vi "Process Flushed Data.vi"(8 "error in":errorcluster, 10 "Flushed elements":T1[](array[typedef]), 11 "Report Generator in":refnum<class "Report Generator.lvclass">) -> (0 "error out":errorcluster, 3 "Report Generator out":refnum<class "Report Generator.lvclass">)   [LabVIEW 2019, in "Report Generator.lvlib" / "Report Generator.lvclass"]
uses:
  Library/Report Generator.lvclass
  C:/Users/Public/Documents/Development/builds/Engine/Engine.lvlibp/Project/Engine.lvclass
  builds/Tools/QDMH.lvlibp/Custom Controls/QDMH Message.ctl
  Library/Report Generator.lvclass/Report Generator.ctl
  builds/Tools/Report.lvlibp/Custom Controls/Report Action.ctl
  builds/Tools/Report.lvlibp/Report.lvclass
  builds/Engine/Engine.lvlibp/Accessors/Read Directory.vi
  builds/Tools/Report.lvlibp/Accessors/Read Open.vi
  builds/Engine/Engine.lvlibp/Accessors/Write Directory.vi
  builds/Tools/QDMH.lvlibp/QDMH.lvclass
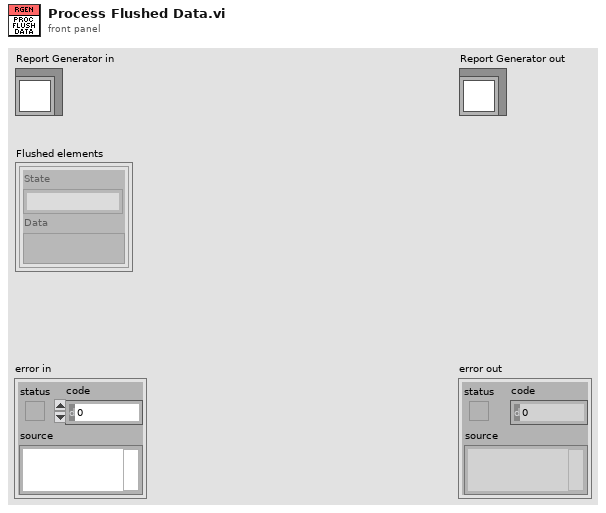
[diagram p1: front panel]
types:
  T1 = typedef "QDMH.lvlibp/QDMH.lvclass/QDMH Message.ctl" = cluster{"State":string, "Data":variant}
  T2 = typedef "Report.lvlibp/Report.lvclass/Report Action.ctl" = enum16{"Create", "Append", "Destroy"}
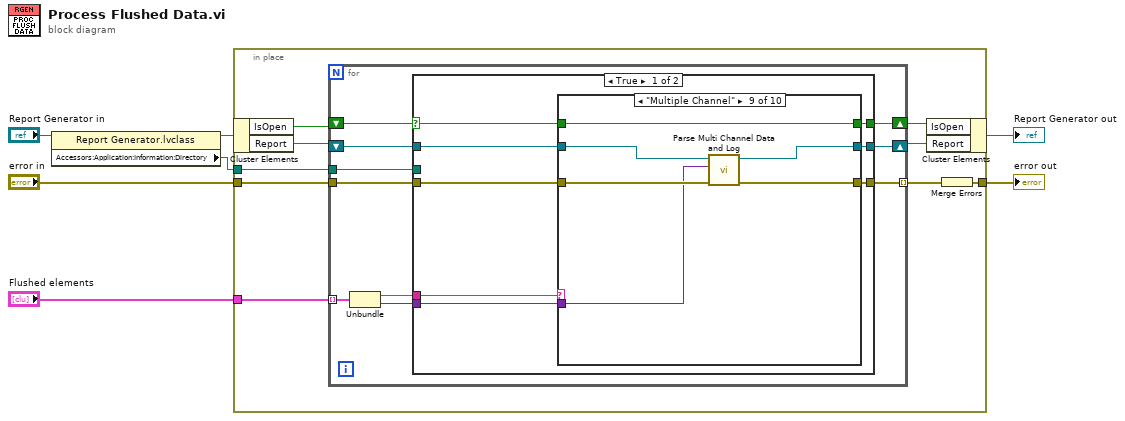
[diagram p0: block diagram]
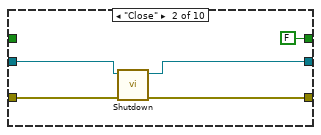
[diagram p3: hidden frame]
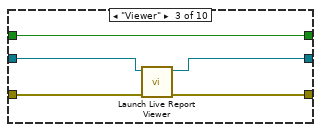
[diagram p4: hidden frame]
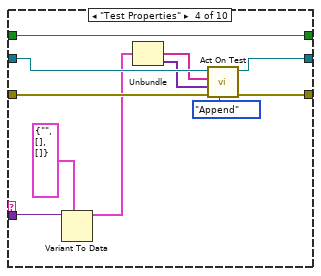
[diagram p5: hidden frame]
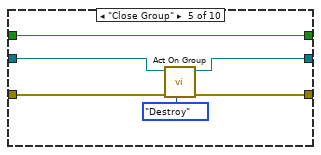
[diagram p6: hidden frame]
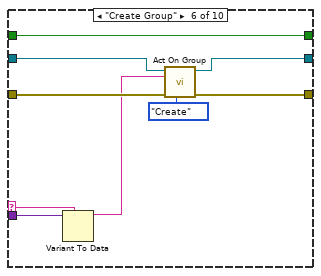
[diagram p7: hidden frame]
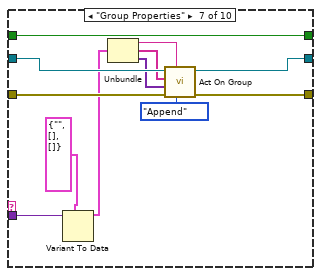
[diagram p8: hidden frame]
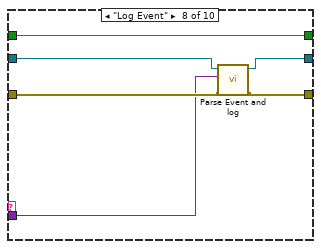
[diagram p9: hidden frame]
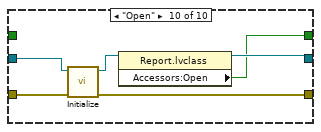
[diagram p10: hidden frame]
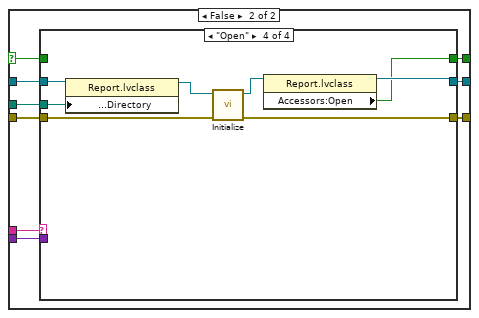
[diagram p11: hidden frame]
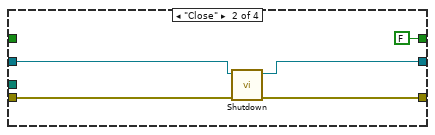
[diagram p13: hidden frame]
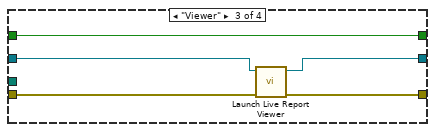
[diagram p14: hidden frame]
diagram:
  n1 = property class="Report Generator.lvclass"(reference="Report Generator in") -> (reference out=w2:refnum<class "Report Generator.lvclass">, "Accessors:Application:Information:Directory"=w1:path)  [unwired: 1 in, 1 out]
  n2 = in-place {
    in-place-border: "Flushed elements" -> [w16]
    in-place-border: "error in" -> [w13]
    in-place-border: [w11] -> w4
    in-place-border: w1 -> [w8]
    n3 = in-place-cluster #1(w2) -> ("IsOpen"=w10:bool, "Report"=w15:refnum<class "Report.lvclass">)
    n4 = for {
      shift-right: [w20] -> w14
      shift-left: w15 -> [w24]
      tunnel: w16 -> [w26] mode=indexing
      tunnel: w13 -> [w22]
      tunnel: [w21] -> w12 mode=indexing
      shift-right: [w19] -> w9
      shift-left: w10 -> [w18]
      tunnel: w8 -> [w17]
      n5 = Unbundle(w26) -> ("State"=w25:string, "Data"=w23:variant)
      n6 = case shown="True" w18 {
        selector: w18 -> [w27 w105]
        tunnel: w25 -> [w34 w112]
        tunnel: w24 -> [w33 w111]
        tunnel: w23 -> [w32 w110]
        tunnel: w22 -> [w31 w109]
        tunnel: [w30 w108] -> w21
        tunnel: [w29 w107] -> w20
        tunnel: [w28 w106] -> w19
        tunnel: w17 -> [_ w104]
        frame True {
          n7 = case shown="\"Multiple Channel\"" w34 {
            selector: w34 -> [_ _ _ _ _ w66 _ _ _ _]
            tunnel: w33 -> [w36 w42 w44 w57 w63 w72 w84 w90 w96 w103]
            tunnel: w32 -> [_ _ _ w52 _ w67 w79 w86 w92 _]
            tunnel: w31 -> [w37 w41 w46 w56 w62 w71 w83 w88 w94 w102]
            tunnel: [w37 w39 w45 w55 w61 w70 w82 w87 w93 w101] -> w30
            tunnel: [w36 w40 w43 w54 w60 w69 w81 w89 w95 w99] -> w29
            tunnel: [w35 FALSE ("Accessors:Open") w47 w58 w64 w73 w85 w91 w97 w98] -> w28
            tunnel: w27 -> [w35 _ w47 w58 w64 w73 w85 w91 w97 _]
            frame Default {
            }
            frame "Close" {
              n8 = call "Shutdown.vi"("error in"=w41, "Report in"=w42) -> ("error out"=w39:errorcluster, "Report out"=w40:refnum<class "Report.lvclass">)  [unwired: 8 in]
            }
            frame "Viewer" {
              n9 = call-dynamic "Launch Live Report Viewer.vi"("error in"=w46, "Report in"=w44) -> ("error out"=w45:errorcluster, "Report out"=w43:refnum<class "Report.lvclass">)  [unwired: 8 in]
            }
            frame "Test Properties" {
              n10 = Variant To Data(type=cluster{string, string[], variant[]} {"", [], []}, Variant=w52) -> (data=w50:cluster{string, string[], variant[]})  [unwired: 1 in, 1 out]
              n11 = Unbundle(w50) -> (w49:string[], w48:variant[])  [unwired: 1 out]
              n12 = call-dynamic "Act On Test.vi"("Report Action"=Report_Action."Append", "error in (no error)"=w56, "Values"=w48, "Parameters"=w49, "Report in"=w57) -> ("error out"=w55:errorcluster, "Report out"=w54:refnum<class "Report.lvclass">)  [unwired: 5 in]
            }
            frame "Close Group" {
              n13 = call-dynamic "Act On Group.vi"("Report Action"=Report_Action."Destroy", "error in (no error)"=w62, "Report in"=w63) -> ("error out"=w61:errorcluster, "Report out"=w60:refnum<class "Report.lvclass">)  [unwired: 7 in]
            }
            frame "Create Group" {
              n14 = Variant To Data(type=w66, Variant=w67) -> (data=w65:string)  [unwired: 1 in, 1 out]
              n15 = call-dynamic "Act On Group.vi"("Report Action"=Report_Action."Create", "Group Name"=w65, "error in (no error)"=w71, "Report in"=w72) -> ("error out"=w70:errorcluster, "Report out"=w69:refnum<class "Report.lvclass">)  [unwired: 6 in]
            }
            frame "Group Properties" {
              n16 = Variant To Data(type=cluster{string, string[], variant[]} {"", [], []}, Variant=w79) -> (data=w77:cluster{string, string[], variant[]})  [unwired: 1 in, 1 out]
              n17 = Unbundle(w77) -> (w76:string, w75:string[], w74:variant[])
              n18 = call-dynamic "Act On Group.vi"("Report Action"=Report_Action."Append", "Group Name"=w76, "error in (no error)"=w83, "Values"=w74, "Parameters"=w75, "Report in"=w84) -> ("error out"=w82:errorcluster, "Report out"=w81:refnum<class "Report.lvclass">)  [unwired: 4 in]
            }
            frame "Log Event" {
              n19 = call "Parse Event and log.vi"("error in"=w88, "Variant"=w86, "Report in"=w90) -> ("error out"=w87:errorcluster, "Report out"=w89:refnum<class "Report.lvclass">)  [unwired: 7 in]
            }
            frame "Multiple Channel" {
              n20 = call "Parse Multi Channel Data and Log.vi"("error in"=w94, "Variant"=w92, "Report in"=w96) -> ("error out"=w93:errorcluster, "Report out"=w95:refnum<class "Report.lvclass">)  [unwired: 7 in]
            }
            frame "Open" {
              n21 = call-dynamic "Initialize.vi"("error in"=w102, "Report in"=w103) -> ("error out"=w101:errorcluster, "Report out"=w100:refnum<class "Report.lvclass">)  [unwired: 8 in]
              n22 = property class="Report.lvclass"(reference=w100) -> (reference out=w99:refnum<class "Report.lvclass">, "Accessors:Open"=w98:bool)  [unwired: 1 in, 1 out]
            }
          }
        }
        frame False {
          n23 = case shown="\"Open\"" w112 {
            tunnel: w111 -> [w114 w120 w122 w128]
            tunnel: w110 -> [_ _ _ _]
            tunnel: w109 -> [w115 w119 w124 w133]
            tunnel: [w115 w117 w123 w132] -> w108
            tunnel: [w114 w118 w121 w130] -> w107
            tunnel: [w113 FALSE ("Accessors:Open") w125 w129] -> w106
            tunnel: w105 -> [w113 _ w125 _]
            tunnel: w104 -> [_ _ _ w126]
            frame Default {
            }
            frame "Close" {
              n24 = call "Shutdown.vi"("error in"=w119, "Report in"=w120) -> ("error out"=w117:errorcluster, "Report out"=w118:refnum<class "Report.lvclass">)  [unwired: 8 in]
            }
            frame "Viewer" {
              n25 = call-dynamic "Launch Live Report Viewer.vi"("error in"=w124, "Report in"=w122) -> ("error out"=w123:errorcluster, "Report out"=w121:refnum<class "Report.lvclass">)  [unwired: 8 in]
            }
            frame "Open" {
              n26 = property class="Report.lvclass"(reference=w128, "Accessors:Application:Information:Directory"=w126) -> (reference out=w127:refnum<class "Report.lvclass">)  [unwired: 1 in, 1 out]
              n27 = call-dynamic "Initialize.vi"("error in"=w133, "Report in"=w127) -> ("error out"=w132:errorcluster, "Report out"=w131:refnum<class "Report.lvclass">)  [unwired: 8 in]
              n28 = property class="Report.lvclass"(reference=w131) -> (reference out=w130:refnum<class "Report.lvclass">, "Accessors:Open"=w129:bool)  [unwired: 1 in, 1 out]
            }
          }
        }
      }
    }
    n29 = in-place-cluster #1("IsOpen"=w9, "Report"=w14) -> (→"Report Generator out":refnum<class "Report Generator.lvclass">)
    n30 = Merge Errors(w12) -> (w11:errorcluster)
  }
  "error out" <- w4
